vi "CreateDAQmxTaskFromP2P.vi"(0 "DAQmx Device Name":tag) -> (1 "task out":refnum<k21>, 2 "Extra Properties":string[][](array[string]))   [LabVIEW 2018]
uses:
  <vilib>/DAQmx/create/channels.llb/DAQmx Create Channel (AI-Current-Basic).vi
  <vilib>/DAQmx/create/channels.llb/DAQmx Create Channel (AI-Temperature-Thermocouple).vi
  <resource>/objmgr/daqmx.rc
panel:
  out "AI.MeasTypes":i32[](array[ring]) items=["Voltage"=10322, "Voltage RMS"=10350, "Current"=10134, "Current RMS"=10351, "More:Voltage:Custom with Excitation"=10323, "More:Bridge (V/V)"=15908, "Frequency"=10181, "Resistance"=10278, "Temperature:Thermocouple"=10303, "Temperature:Thermistor"=10302, "Temperature:RTD"=10301, "Temperature:Built-in Sensor"=10311, "Strain Gage"=10300, "Rosette Strain Gage"=15980, "Position:LVDT"=10352, "Position:RVDT"=10353, "Position:Eddy Current Proximity Probe"=14835, "Accelerometer"=10356, "Acceleration:Charge"=16104, "Acceleration:4 Wire DC Voltage"=16106, "Velocity:IEPE Sensor"=15966, "Force:Bridge"=15899, "Force:IEPE Sensor"=15895, "Pressure:Bridge"=15902, "Sound Pressure:Microphone"=10354, "Torque:Bridge"=15905, "TEDS Sensor"=12531, "Charge"=16105]
  out "Channels":refnum<k21>[](array[refnum])
  out "Input Type":string
  out "Array In":string[][](array[string])
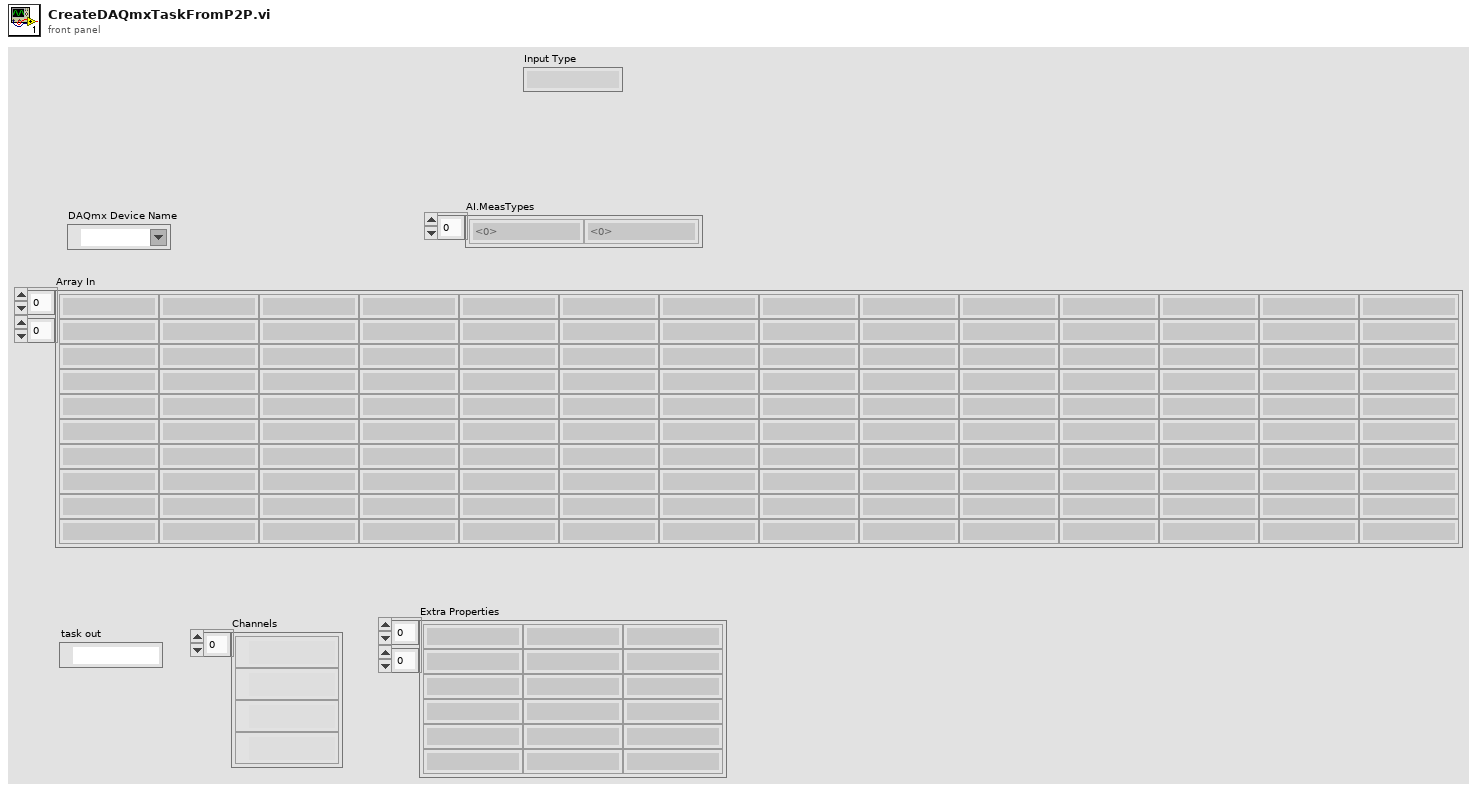
[diagram p1: front panel]
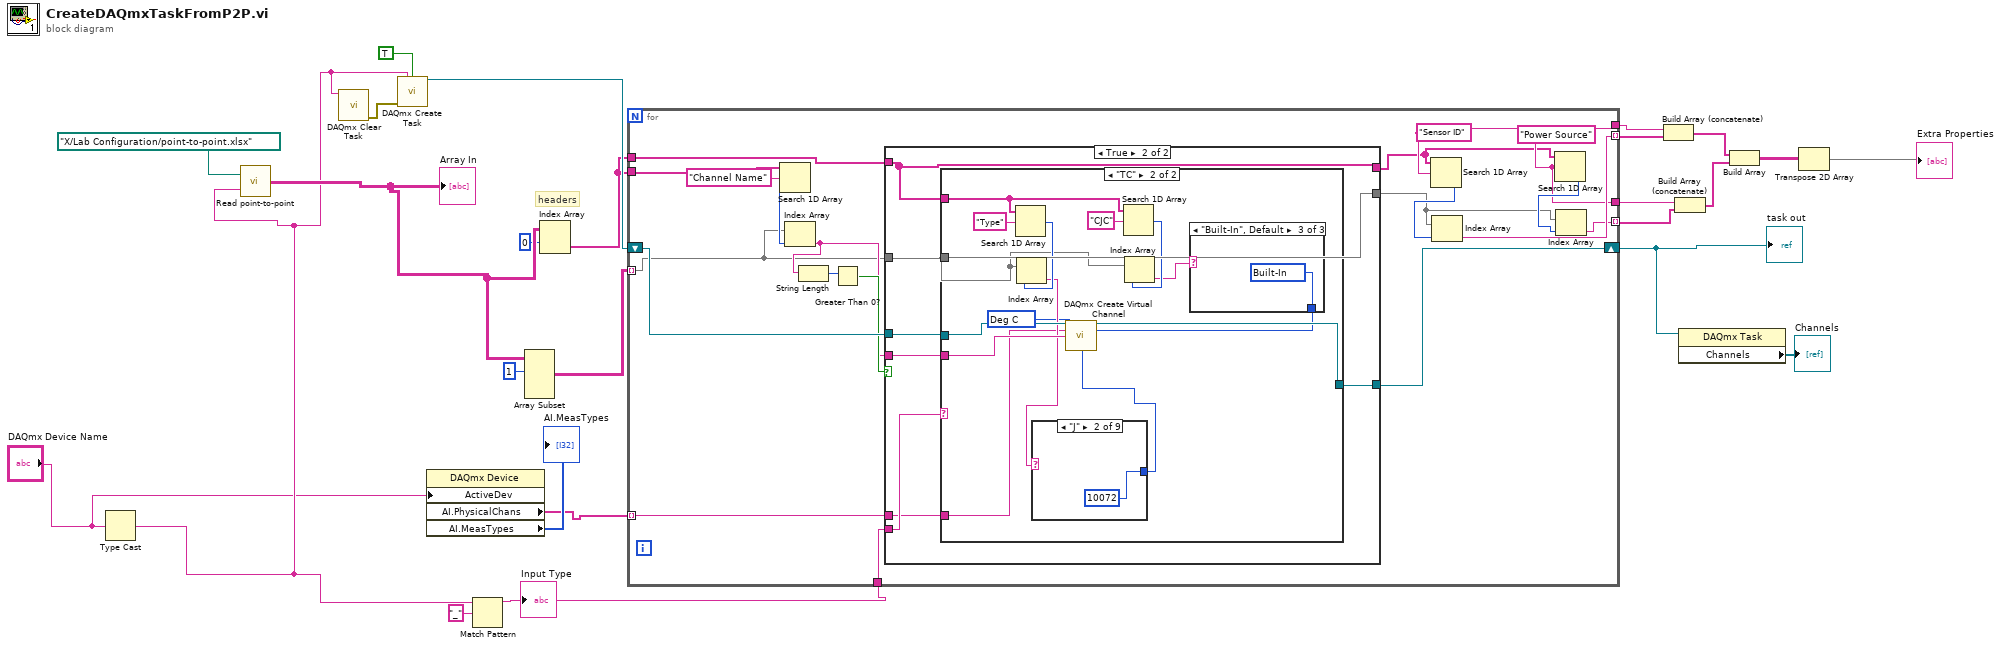
[diagram p0: block diagram]
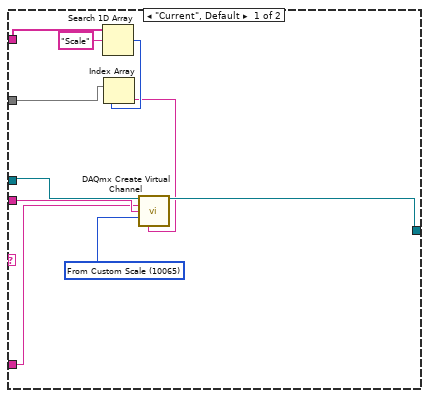
[diagram p3: hidden frame]
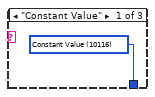
[diagram p4: hidden frame]
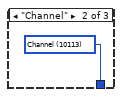
[diagram p5: hidden frame]
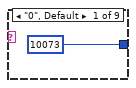
[diagram p6: hidden frame]
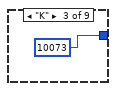
[diagram p7: hidden frame]
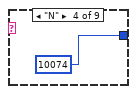
[diagram p8: hidden frame]
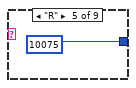
[diagram p9: hidden frame]
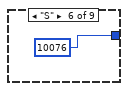
[diagram p10: hidden frame]
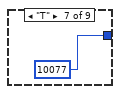
[diagram p11: hidden frame]
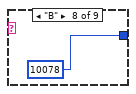
[diagram p12: hidden frame]
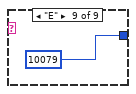
[diagram p13: hidden frame]
diagram:
  # "headers"
  n1 = Type Cast(x="DAQmx Device Name") -> (*(type *) &x=w4:string)  [unwired: 1 in]
  n2 = call "Read point-to-point.vi"("Worksheet Name"=w4, "Path"=path "X:/Lab Configuration/point-to-point.xlsx") -> ("Array Out"=w19:string[][])
  "Array In" <- w19
  n3 = call <vilib>:"DAQmx Clear Task.vi"("task in"=w4) -> ("error out"=w22:errorcluster)  [unwired: 14 in]
  n4 = call <vilib>:"DAQmx Create Task.vi"("new task name"=w4, "auto cleanup"=TRUE, "error in"=w22) -> ("task out"=w24:refnum<k21>)  [unwired: 11 in, 1 out]
  n5 = property class="DAQmx Device"("ActiveDev"="DAQmx Device Name") -> ("AI.PhysicalChans"=w1:tag[], "AI.MeasTypes"=→"AI.MeasTypes":i32[])  [unwired: 2 in, 2 out]
  n6 = Match Pattern(string=w4, regular expression="_") -> (before substring=w8:string)  [unwired: 1 in, 3 out]
  "Input Type" <- w8
  n7 = Array Subset(array=w19, index (row)=1 ("index")) -> (w20:string[][])  [unwired: 3 in]
  n8 = Index Array(array=w19, index (row)=0) -> (element=w7:string[])  [unwired: 1 in]
  n9 = for {
    tunnel: w20 -> [w30] mode=indexing
    shift-right: [w44] -> w6
    shift-left: w24 -> [w45]
    tunnel: w7 -> [w35]
    tunnel: [w37] -> w16 mode=indexing
    tunnel: [w36] -> w17
    tunnel: [w33] -> w14 mode=indexing
    tunnel: [w32] -> w15
    tunnel: w8 -> [w31]
    tunnel: w7 -> [w29]
    tunnel: w1 -> [w26] mode=indexing
    w32 = "Power Source" ("element")
    w36 = "Sensor ID" ("element")
    n10 = Search 1D Array(1D array=w35, element="Channel Name") -> (index of element=w39:i32)  [unwired: 1 in]
    n11 = Index Array(array=w30, index=w39) -> (element=w41:string)
    n12 = String Length(string=w41) -> (length=w43:i32)
    n13 = Greater Than 0?(x=w43) -> (x > 0?=w42:bool)
    n14 = case shown="True" w42 {
      tunnel: w45 -> [w48 w55]
      tunnel: [w48 w54] -> w44
      tunnel: w41 -> [_ w53]
      tunnel: w31 -> [_ w52]
      tunnel: w30 -> [w46 w50]
      tunnel: w29 -> [w47 w51]
      tunnel: [w47 w51] -> w28
      tunnel: [w46 w50] -> w27
      tunnel: w26 -> [_ w49]
      frame False {
      }
      frame True {
        n15 = case shown="\"TC\"" w52 {
          tunnel: w55 -> [w65 w80]
          tunnel: [w64 w79] -> w54
          tunnel: w53 -> [w63 w78]
          tunnel: w50 -> [w61 w68]
          tunnel: w51 -> [w59 w69]
          tunnel: w49 -> [w56 w72]
          frame "Current", Default {
            w62 = 10065 items=["Amps"=10342, "From Custom Scale"=10065] ("units")
            n16 = Search 1D Array(1D array=w59, element="Scale") -> (index of element=w58:i32)  [unwired: 1 in]
            n17 = Index Array(array=w61, index=w58) -> (element=w57:string)
            n18 = call-poly <vilib>:"DAQmx Create Virtual Channel.vi"("task in"=w65, "physical channels"=w56, "name to assign"=w63, "units"=w62, "custom scale name"=w57) -> ("task out"=w64:refnum<k21>)  [unwired: 9 in, 1 out]
          }
          frame "TC" {
            w74 = 10143 items=["Deg C"=10143, "Deg F"=10144, "Kelvins"=10325, "Deg R"=10145, "From Custom Scale"=10065] ("units")
            n19 = Search 1D Array(1D array=w69, element="Type") -> (index of element=w76:i32)  [unwired: 1 in]
            n20 = Index Array(array=w68, index=w76) -> (element=w75:string)
            n21 = case shown="\"J\"" w75 {
              tunnel: [10073 10072 10073 10074 10075 10076 10077 10078 10079] -> w73
              frame "0", Default {
              }
              frame "J" {
              }
              frame "K" {
              }
              frame "N" {
              }
              frame "R" {
              }
              frame "S" {
              }
              frame "T" {
              }
              frame "B" {
              }
              frame "E" {
              }
            }
            n22 = Search 1D Array(1D array=w69, element="CJC") -> (index of element=w71:i32)  [unwired: 1 in]
            n23 = Index Array(array=w68, index=w71) -> (element=w67:string)
            n24 = case shown="\"Built-In\", Default" w67 {
              tunnel: [w81 w82 w83] -> w66
              frame "Constant Value" {
                w81 = 10116 items=["Built-In"=10200, "Constant Value"=10116, "Channel"=10113] ("cjc source")
              }
              frame "Channel" {
                w82 = 10113 items=["Built-In"=10200, "Constant Value"=10116, "Channel"=10113] ("cjc source")
              }
              frame "Built-In", Default {
                w83 = 10200 items=["Built-In"=10200, "Constant Value"=10116, "Channel"=10113] ("cjc source")
              }
            }
            n25 = call-poly <vilib>:"DAQmx Create Virtual Channel.vi"("task in"=w80, "physical channels"=w72, "cjc source"=w66, "name to assign"=w78, "units"=w74, "thermocouple type"=w73) -> ("task out"=w79:refnum<k21>)  [unwired: 8 in, 1 out]
          }
        }
      }
    }
    n26 = Search 1D Array(1D array=w28, element=w36) -> (index of element=w38:i32)  [unwired: 1 in]
    n27 = Index Array(array=w27, index=w38) -> (element=w37:string)
    n28 = Search 1D Array(1D array=w28, element=w32) -> (index of element=w34:i32)  [unwired: 1 in]
    n29 = Index Array(array=w27, index=w34) -> (element=w33:string)
  }
  "task out" <- w6
  n30 = Build Array (concatenate)(w17, w16) -> (w13:string[])
  n31 = Build Array (concatenate)(w15, w14) -> (w12:string[])
  n32 = property class="DAQmx Task"(reference=w6) -> ("Channels"=→"Channels":refnum<k21>[])  [unwired: 1 in, 2 out]
  n33 = Build Array(w13, w12) -> (w11:string[][])
  n34 = Transpose 2D Array(2D array=w11) -> (transposed array=→"Extra Properties":string[][])
